vi "test_from_photonvision_get_target_from_id.vi"() -> ()   [LabVIEW 2019]
uses:
  <vilib>/Rock Robotics/WPI/ThirdParty/PhotonVisionLib/TypeDef/PhotonTrackedTargetType.ctl
  <vilib>/Rock Robotics/WPI/ThirdParty/PhotonVisionLib/TypeDef/TargetCornerType.ctl
  <vilib>/Rock Robotics/WPI/ThirdParty/JAS_Junk/TrajLib/TypeDef/TRANSFORM3D.ctl
  <vilib>/Rock Robotics/WPI/ThirdParty/JAS_Junk/TrajLib/TypeDef/TRANSLATION3D.ctl
  <vilib>/Rock Robotics/WPI/ThirdParty/JAS_Junk/TrajLib/TypeDef/ROTATION3D.ctl
  <vilib>/Rock Robotics/WPI/ThirdParty/JAS_Junk/TrajLib/TypeDef/QUATERNION.ctl
  <vilib>/Rock Robotics/WPI/ThirdParty/PhotonVisionLib/PhotonVisionLib.lvlib
  <vilib>/Rock Robotics/WPI/ThirdParty/JAS_Junk/TrajLib/Trajectory_Library.lvlib
panel:
  out "HasTargets":bool
  in  "CameraName":string="main"
  out "Target Index":i32
  out "Found Target?":bool
  out "Found PhotonTrackedTarget":T1={"Yaw"=0.0, "Pitch"=0.0, "Area"=0.0, "Skew"=0.0, "MinAreaRectCorners"=[], "BestCameraToTarget"={"TRANSLATION3D"={"X"=0.0, "Y"=0.0, "Z"=0.0}, "ROTATION3D"={"Q_quaternion"={"R"=1.0, "V"=[0.0, 0.0, 0.0]}}, "XF"=FALSE}, "FiiducialId"=0, "AltCameraToTarget"={"TRANSLATION3D"={"X"=0.0, "Y"=0.0, "Z"=0.0}, "ROTATION3D"={"Q_quaternion"={"R"=0.0, "V"=[0.0, 0.0, 0.0]}}, "XF"=FALSE}, "PoseAmbiguity"=0.0, "DetectedCorners"=[]} {"AltCameraToTarget"."TRANSLATION3D"."Z" format="%14.3f"; "AltCameraToTarget"."TRANSLATION3D"."Y" format="%14.3f"; "AltCameraToTarget"."TRANSLATION3D"."X" format="%14.3f"; "BestCameraToTarget"."TRANSLATION3D"."Z" format="%14.3f"; "BestCameraToTarget"."TRANSLATION3D"."Y" format="%14.3f"; "BestCameraToTarget"."TRANSLATION3D"."X" format="%14.3f"}
  in  "ID":i32
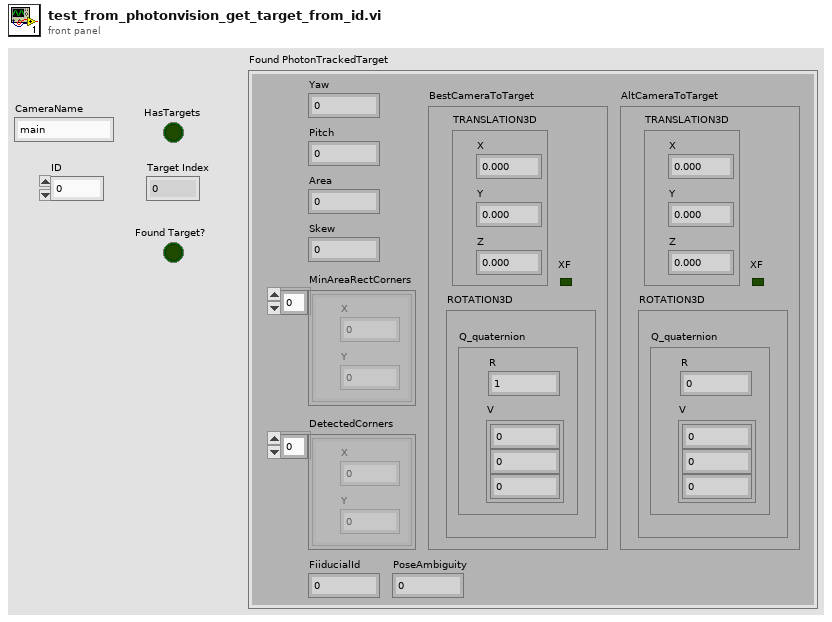
[diagram p1: front panel]
types:
  T1 = typedef "PhotonVisionLib.lvlib/PhotonTrackedTargetType.ctl" = cluster{"Yaw":dbl, "Pitch":dbl, "Area":dbl, "Skew":dbl, "MinAreaRectCorners":T2[], "BestCameraToTarget":T3, "FiiducialId":i32, "AltCameraToTarget":T3, "PoseAmbiguity":dbl, "DetectedCorners":T2[]}
  T2 = typedef "PhotonVisionLib.lvlib/TargetCornerType.ctl" = cluster{"X":dbl, "Y":dbl}
  T3 = typedef "Trajectory_Library.lvlib/TRANSFORM3D.ctl" = cluster{"TRANSLATION3D":T4, "ROTATION3D":T5, "XF":bool}
  T4 = typedef "Trajectory_Library.lvlib/TRANSLATION3D.ctl" = cluster{"X":dbl, "Y":dbl, "Z":dbl}
  T5 = typedef "Trajectory_Library.lvlib/ROTATION3D.ctl" = cluster{"Q_quaternion":T6}
  T6 = typedef "Trajectory_Library.lvlib/QUATERNION.ctl" = cluster{"R":dbl, "V":dbl[]}
  T7 = typedef "PhotonVisionLib.lvlib/PhotonPipelineResultType.ctl" = cluster{"TargetCount":i32, "Latency_MilliSec":dbl, "Targets":T1[], "TimeStampSec":dbl}
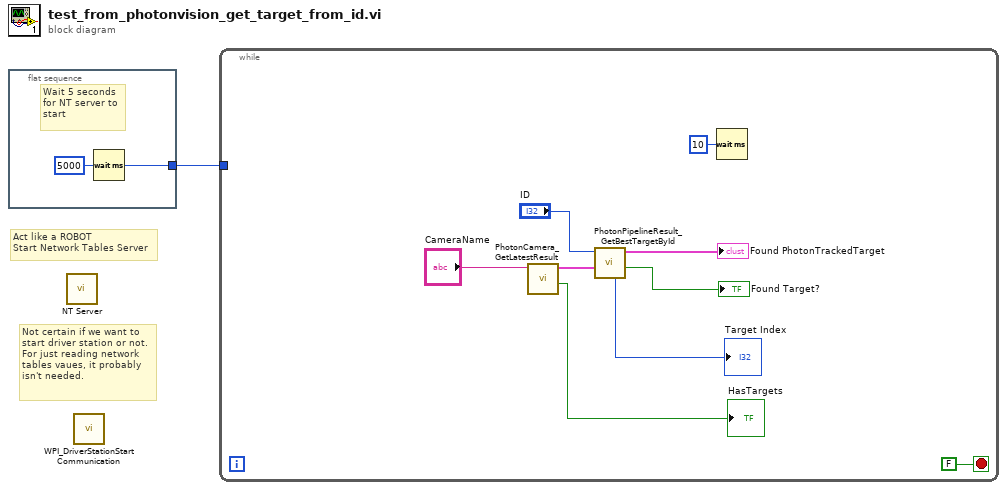
[diagram p0: block diagram]
diagram:
  # "Not certain if we want to\nstart driver station or not.\nFor just reading network\ntables vaues, it probably\nisn't needed."
  # "Act like a ROBOT\nStart Network Tables Server"
  n1 = flat-sequence {
    tunnel: [w2] -> w1
    frame #0 {
      # "Wait 5 seconds\nfor NT server to\nstart"
      n2 = Wait (ms)(milliseconds to wait=u32 5000) -> (millisecond timer value=w2:u32)
    }
  }
  n3 = call <vilib>:"NT Server.vi"() -> ()  [unwired: 12 in]
  n4 = call <vilib>:"WPI_DriverStationStart Communication.vi"() -> ()  [unwired: 12 in]
  n5 = while {
    tunnel: w1 -> [_]
    stop <- FALSE stop-if-true
    n6 = call <vilib>:"PhotonCamera_GetLatestResult.vi"("CameraName"="CameraName") -> ("HasTargets"=→"HasTargets":bool, "PipelineResult"=w5:T7)  [unwired: 9 in]
    n7 = call <vilib>:"PhotonPipelineResult_GetBestTargetById.vi"("PhotonPipelineResult"=w5, "FiducialId"="ID") -> ("Target Found"=→"Found Target?":bool, "PhotonTrackedTarget"=→"Found PhotonTrackedTarget":T1, "Target Index"=→"Target Index":i32)  [unwired: 7 in]
    n8 = Wait (ms)(milliseconds to wait=u32 10) -> ()  [unwired: 1 out]
  }
